vi "Arcade with Deadband.vi"(4 "Turning Deadband":dbl, 5 "Speed Deadband":dbl, 7 "Square Inputs":bool=TRUE, 8 "Turning Rate":dbl=1.0, 9 "Speed Rate":dbl=1.0, 10 "Turning Setpoint":dbl, 11 "Speed Setpoint":dbl) -> (2 "Right Motor Value":dbl, 3 "Left Motor Value":dbl)   [LabVIEW 2017]
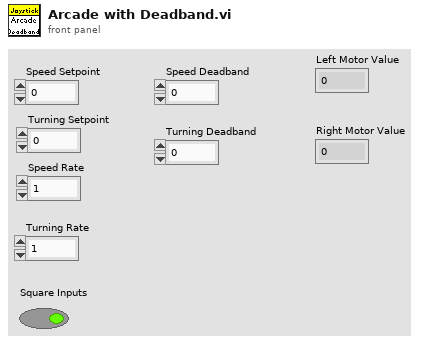
[diagram p1: front panel]
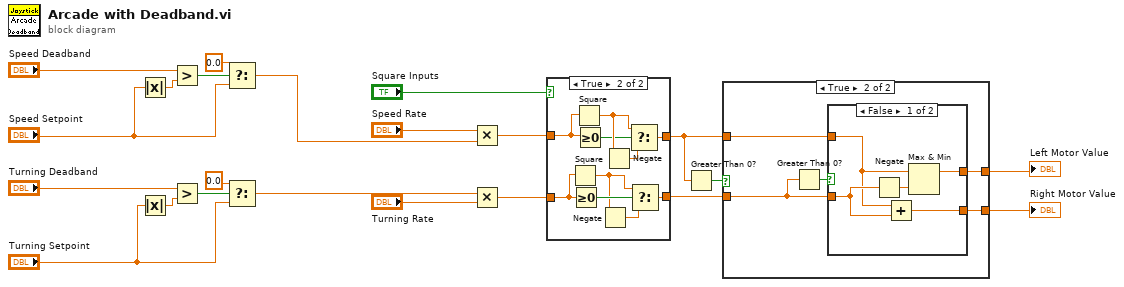
[diagram p0: block diagram]
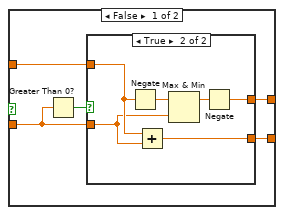
[diagram p2: hidden frame]
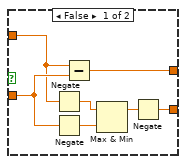
[diagram p3: hidden frame]
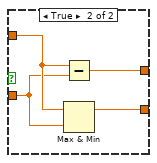
[diagram p4: hidden frame]
diagram:
  n1 = Absolute Value(x="Speed Setpoint") -> (abs(x)=w11:dbl)
  n2 = Absolute Value(x="Turning Setpoint") -> (abs(x)=w5:dbl)
  n3 = Greater?(x="Speed Deadband", y=w11) -> (0:w10:bool)
  n4 = Greater?(x="Turning Deadband", y=w5) -> (0:w6:bool)
  n5 = Select(t=0.0, s=w10, f="Speed Setpoint") -> (s? t:f=w7:dbl)
  n6 = Select(t=0.0, s=w6, f="Turning Setpoint") -> (s? t:f=w2:dbl)
  n7 = Multiply(x="Speed Rate", y=w7) -> (x*y=w17:dbl)
  n8 = Multiply(x=w2, y="Turning Rate") -> (x*y=w15:dbl)
  n9 = case shown="True" "Square Inputs" {
    tunnel: [w23 w34] -> w20
    tunnel: [w24 w33] -> w21
    tunnel: w15 -> [w23 w32]
    tunnel: w17 -> [w24 w31]
    frame False {
    }
    frame True {
      n10 = Square(x=w32) -> (x^2=w29:dbl)
      n11 = Greater Or Equal To 0?(x=w32) -> (x >= 0?=w30:bool)
      n12 = Square(x=w31) -> (x^2=w26:dbl)
      n13 = Greater Or Equal To 0?(x=w31) -> (x >= 0?=w25:bool)
      n14 = Negate(x=w29) -> (-x=w28:dbl)
      n15 = Negate(x=w26) -> (-x=w27:dbl)
      n16 = Select(t=w26, s=w25, f=w27) -> (s? t:f=w33:dbl)
      n17 = Select(t=w29, s=w30, f=w28) -> (s? t:f=w34:dbl)
    }
  }
  n18 = Greater Than 0?(x=w21) -> (x > 0?=w22:bool)
  n19 = case shown="True" w22 {
    tunnel: w20 -> [w38 w56]
    tunnel: w21 -> [w37 w55]
    tunnel: [w36 w54] -> w14
    tunnel: [w35 w53] -> w13
    frame False {
      n20 = Greater Than 0?(x=w38) -> (x > 0?=w39:bool)
      n21 = case shown="True" w39 {
        tunnel: w38 -> [w46 w48]
        tunnel: w37 -> [w44 w49]
        tunnel: [w40 w50] -> w36
        tunnel: [w41 w47] -> w35
        frame False {
          n22 = Negate(x=w44) -> (-x=w45:dbl)
          n23 = Negate(x=w46) -> (-x=w43:dbl)
          n24 = Subtract(x=w44, y=w46) -> (x-y=w40:dbl)
          n25 = Max & Min(x=w45, y=w43) -> (max(x,y)=w42:dbl)  [unwired: 1 out]
          n26 = Negate(x=w42) -> (-x=w41:dbl)
        }
        frame True {
          n27 = Negate(x=w49) -> (-x=w52:dbl)
          n28 = Add(x=w49, y=w48) -> (x+y=w47:dbl)
          n29 = Max & Min(x=w52, y=w48) -> (max(x,y)=w51:dbl)  [unwired: 1 out]
          n30 = Negate(x=w51) -> (-x=w50:dbl)
        }
      }
    }
    frame True {
      n31 = Greater Than 0?(x=w56) -> (x > 0?=w57:bool)
      n32 = case shown="False" w57 {
        tunnel: w56 -> [w62 w64]
        tunnel: w55 -> [w59 w65]
        tunnel: [w60 w63] -> w54
        tunnel: [w58 w66] -> w53
        frame False {
          n33 = Negate(x=w62) -> (-x=w61:dbl)
          n34 = Add(x=w59, y=w62) -> (x+y=w58:dbl)
          n35 = Max & Min(x=w59, y=w61) -> (max(x,y)=w60:dbl)  [unwired: 1 out]
        }
        frame True {
          n36 = Subtract(x=w65, y=w64) -> (x-y=w63:dbl)
          n37 = Max & Min(x=w65, y=w64) -> (max(x,y)=w66:dbl)  [unwired: 1 out]
        }
      }
    }
  }
  "Right Motor Value" <- w13
  "Left Motor Value" <- w14
